vi "TRIG_PREF_AIGL.vi"(0 "VISA IN":refnum<visa-resource-name>, 5 "error in":errorcluster, 7 "Global":bool) -> (14 "VISA Out":refnum<visa-resource-name>, 19 "error out":errorcluster)   [LabVIEW 2018, in "PNA-X.lvlib"]
doc: "TRIGger:PREFerence:AIGLobal <bool> \n(Read-Write) Sets the External Trigger OUT behavior to either Global or Channel. Learn more. \nThis command will cause the PNA to Preset. \nThis setting remains until changed again using this command, or until the hard drive is changed or \nreformatted. \nTo send this command using the PNA front panel, open the GPIB Command Processor Console, then \ntype either of the following examples at the command prompt. Then type the Query Syntax and press \nenter to be sure the PNA took the command. \nParameters \n<bool> Choose from: \nON (or 1) - External I/O Trig properties apply to ALL channels (Global) \nOFF (or 0) - External I/O Trig properties apply to each channel independently. \nExamples TRIG:PREF:AIGL 1 \ntrigger:preference:aiglobal 0 \nQuery Syntax TRIGger:PREFerence:AIGLobal? \nReturn Type Boolean \nDefault 1 - E836xB and PNA-L models \n0 - PNA-X models \nTRIGger[:SEQuence]:LEVel <char> - Superseded \n1895\n\nThis command is replaced with CONTrol:SIGNal \n(Read-Write) Triggers either on a High or Low level trigger signal. This setting only has an effect \nwhen TRIG:SOURce EXTernal is selected. \nParameters \n<char> Choose from: \nHIGH - analyzer triggers on TTL High \nLOW - analyzer triggers on TTL Low \nExamples TRIG:LEV HIGH \ntrigger:sequence:level low \nQuery Syntax TRIGger[:SEQuence]:LEVel? \nReturn Type Character \nDefault LOW \nTRIGger[:SEQuence]:SCOPe <char> \n(Read-Write) Specifies whether a trigger signal is sent to all channels or only the current channel. \nSee Triggering the PNA using SCPI. \nParameters \n<char> Choose from: \nALL - trigger signal is sent to all channels. Also sets SENS:SWEep:TRIG:POINt \nOFF on ALL channels. \nCURRent - trigger signal is sent to only one channel at a time. With each trigger \nsignal, the channel is incremented to the next triggerable channel. \nExamples TRIG:SCOP ALL \ntrigger:sequence:scope current \nQuery Syntax TRIGger[:SEQuence]:SCOPe? \nReturn Type Character \nDefault ALL \nTRIGger[:SEQuence]:SOURce <char> \n1896\n\n(Read-Write) Sets the source of the sweep trigger signal. This command is a super-set of \nINITiate:CONTinuous, which can NOT set the source to External. To configure external triggering, \nsee CONTrol:SIGNal. \nSee Triggering the PNA using SCPI. \nParameters \n<char> Choose from: \nEXTernal - external (rear panel) source. \nIMMediate - internal source sends continuous trigger signals \nMANual - sends one trigger signal when manually triggered from the front panel or \nINIT:IMM is sent. \nExamples TRIG:SOUR EXT \ntrigger:sequence:source immediate \nQuery Syntax TRIGger[:SEQuence]:SOURce? \nReturn Type Character \nDefault IMMediate"
uses:
  PNA-X.lvlib
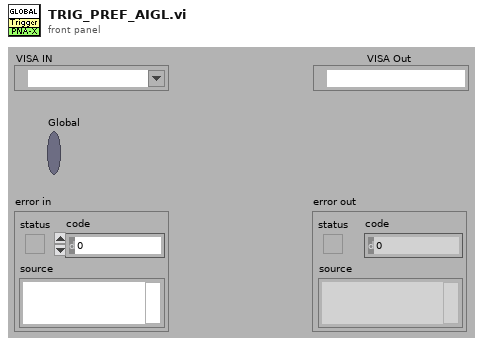
[diagram p1: front panel]
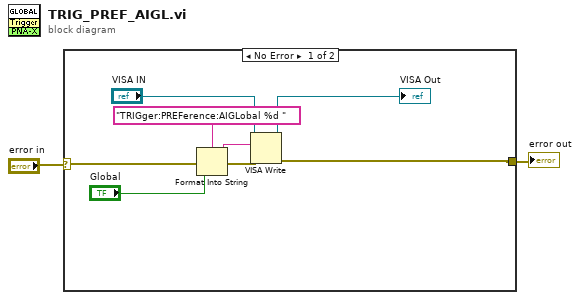
[diagram p0: block diagram]
diagram:
  n1 = case shown="No Error" "error in" {
    selector: "error in" -> [w10 w11]
    tunnel: [w5 w11] -> w1
    frame No Error {
      n2 = Format Into String(format string="TRIGger:PREFerence:AIGLobal %d " ("Cmdline"), error in=w10, "Global") -> (resulting string=w8:string, error out=w9:errorcluster)  [unwired: 1 in]
      n3 = VISA Write(VISA resource name="VISA IN", write buffer=w8, error in (no error)=w9) -> (VISA resource name out=→"VISA Out":refnum<visa-resource-name>, error out=w5:errorcluster)  [unwired: 1 out]
    }
    frame Error {
    }
  }
  "error out" <- w1
